vi "Main Loop.vi"(8 "error in (no error)":errorcluster, 10 "Chart Notifier":refnum<notifier>, 11 "Message Queues":T1) -> (0 "error out":errorcluster)   [LabVIEW 2018, in "OPC UA.lvlib" / "OPC UA Module Engine.lvlib"]
uses:
  OPC UA Module Engine.lvlib
  Message Queues.ctl
  support/Message Queue/Message Cluster.ctl
  OPC Display Cluster.ctl
  OPC Module Config.ctl
  Scale Module Folder/Measure Instrument/State Enum.ctl
  <vilib>/Utility/miscctls.llb/LVPoint32TypeDef.ctl
  OPC Settings.ctl
  Variable Data Cluster.ctl
  <vilib>/OPCUA/controls/NodeId.ctl
  <vilib>/OPCUA/controls/OPC UA StatusCode.ctl
  <vilib>/OPCUA/controls/Subscription ID.ctl
  <vilib>/OPCUA/controls/OPC UA Client Refnum.ctl
  <vilib>/OPCUA/controls/Subscription Data Change.ctl
  <vilib>/OPCUA/controls/Data Type.ctl
  <vilib>/Platform/TimedLoop/XDataNode/timing_clust.ctl
  <vilib>/Platform/TimedLoop/XDataNode/nitl_modes.ctl
  <vilib>/Platform/TimedLoop/XDataNode/wakeup.ctl
  Tag VIs/Tag FGV Operation Enum.ctl
  support/Message Queue/Enqueue Message (Single).vi
  <vilib>/Platform/TimedLoop/XDataNode/XDataNode.xnode
  Scale Module Folder/Measure Instrument/Scale Module Engine.lvlib
  OPC UA.lvlib
  <vilib>/Platform/TimedLoop/XDataNode/XDNodeRunTimeDep.lvlib
  support/Support Library.lvlib
  Shared Variables/Dynamic Shared Variables.lvlib
  support/Message Queue/Message Queue.lvlib
panel:
  out "Period (s)":dbl format="%_4g"
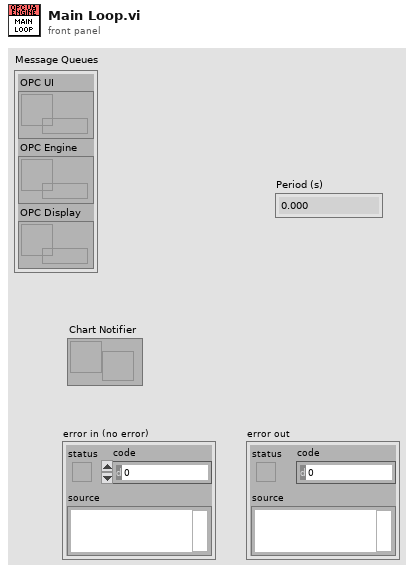
[diagram p1: front panel]
types:
  T1 = typedef "OPC UA.lvlib/Message Queues.ctl" = cluster{"OPC UI":refnum<queue>, "OPC Engine":refnum<queue>, "OPC Display":refnum<queue>}
  T2 = typedef "OPC UA.lvlib/OPC Display Cluster.ctl" = cluster{"URL":string, "Cycle":i32, "Updating":bool}
  T3 = typedef "XDNodeRunTimeDep.lvlib/timing_clust.ctl" = cluster{"Expected End [f-1]":u64, "Actual End [f-1]":u64, "Finished Late? [f-1]":bool, "Expected End [i-1]":u64, "Actual End [i-1]":u64, "Finished Late? [i-1]":bool, "Expected Start [i]":u64, "Actual Start [i]":u64, "Expected Start [f]":u64, "Actual Start [f]":u64, "Source Name":string, "Structure Name":string, "Period":i64, "Deadline":i64, "Offset":i64, "Start":i64, "Priority":i32, "Timeout":i32, "Mode":T4, "Wakeup Reason":T5, "Error":errorcluster, "Source Type":string, "Secondary Source Type":string, "Global End Time":u64, "Global Start Time":u64, "Frame Duration":u64, "Iteration Duration":u64, "Assigned CPU":i32, "I/O Scan Engine Mode":u32}
  T4 = typedef "XDNodeRunTimeDep.lvlib/nitl_modes.ctl" = enum32{"No Change", "Process missed periods, maintain original phase", "Discard missed periods, maintain original phase", "Process missed periods, ignore original phase", "Discard missed periods, ignore original phase"}
  T5 = typedef "XDNodeRunTimeDep.lvlib/wakeup.ctl" = enum32{"Normal", "Aborted", "Asynchronous wakeup", "Timing source error", "Timed loop error", "Timeout"}
  T6 = cluster{"enable? (F)":bool, "name":string, "alarm on":bool, "priority":u32, "ack type":enum16{"Auto", "User", "None", "Each Occurrence"}, "area":string, "description":string, "log? (T)":bool}
  T7 = typedef "Tag FGV Operation Enum.ctl" = enum16{"Init", "Set Notification Queue", "Create Tag", "Commit", "Write Tag (Numeric)", "Write Tag (Boolean)", "Read All Tags", "Read One Tag", "Delete Tag Category", "Set Alarm Parameters (Numeric)", "Set Alarm Parameters (Boolean)", "Enable All Alarms", "Disable All Alarms", "Delete All Tags", "Read Alarms", "Ack Alarm", "Read Alarm Parameters (Numeric)", "Read Alarm Parameters (Boolean)"}
  T8 = enum32{"u32BitField", "bool", "double", "string", "int8", "uint8", "int16", "uint16", "int32", "uint32", "int64", "uint64", "single", "double waveform", "int16 waveform", "array of boolean", "array of int8", "array of uint8", "array of int16", "array of uint16", "array of int32", "array of uint32", "array of int64", "array of uint64", "array of single", "array of double", "array of double waveform", "array of int16 waveform", "array of string", "variant", "timestamp", "fixed point", "custom"}
  T9 = typedef "Scale Module.lvlib/Scale Module Engine.lvlib/State Enum.ctl" = enum16{"Measuring", "Idle"}
  T10 = typedef "OPC UA.lvlib/OPC Settings.ctl" = cluster{"Cycle Period":dbl, "server endpoint URL":string, "security policy":cluster{"message mode":enum16{"None", "Sign", "Sign and Encrypt"}, "security":enum16{"Basic256", "Basic128Rsa15"}}, "Trust Any Server":bool}
  T11 = typedef "OPC UA.lvlib/OPC Module Config.ctl" = cluster{"State":T9, "GUID":string, "Drop Coords":T12, "Configuration":T10, "First Iteration":bool, "Data":cluster{"Object Name":string, "Variable Array":T13[]}[], "Process Name":string, "Load Count":i32, "Log Started":bool, "subscription ID out":T16, "OPC UA client refnum out":T17, "Event Registration Refnum":refnum<event-registration>, "Start Time":timestamp, "Current Time":timestamp}
  T12 = typedef "LVPoint32TypeDef.ctl" = cluster{"Horizontal":i32, "Vertical":i32}
  T13 = typedef "OPC UA.lvlib/Variable Data Cluster.ctl" = cluster{"node ID":T14, "browse name":string, "status":T15, "timestamp":timestamp, "value ":variant}
  T14 = typedef "NodeId.ctl" = string
  T15 = typedef "OPC UA StatusCode.ctl" = u32
  T16 = typedef "Subscription ID.ctl" = u32
  T17 = typedef "OPC UA Client Refnum.ctl" = refnum<k21>
  T18 = cluster{"Object Name":string, "Variable Array":T13[]}[]
  T19 = cluster{"Object Name":string, "Variable Array":T13[]}
  T20 = typedef "Support Library.lvlib/Message Queue.lvlib/Message Cluster.ctl" = cluster{"Message":string, "Message Data":variant}
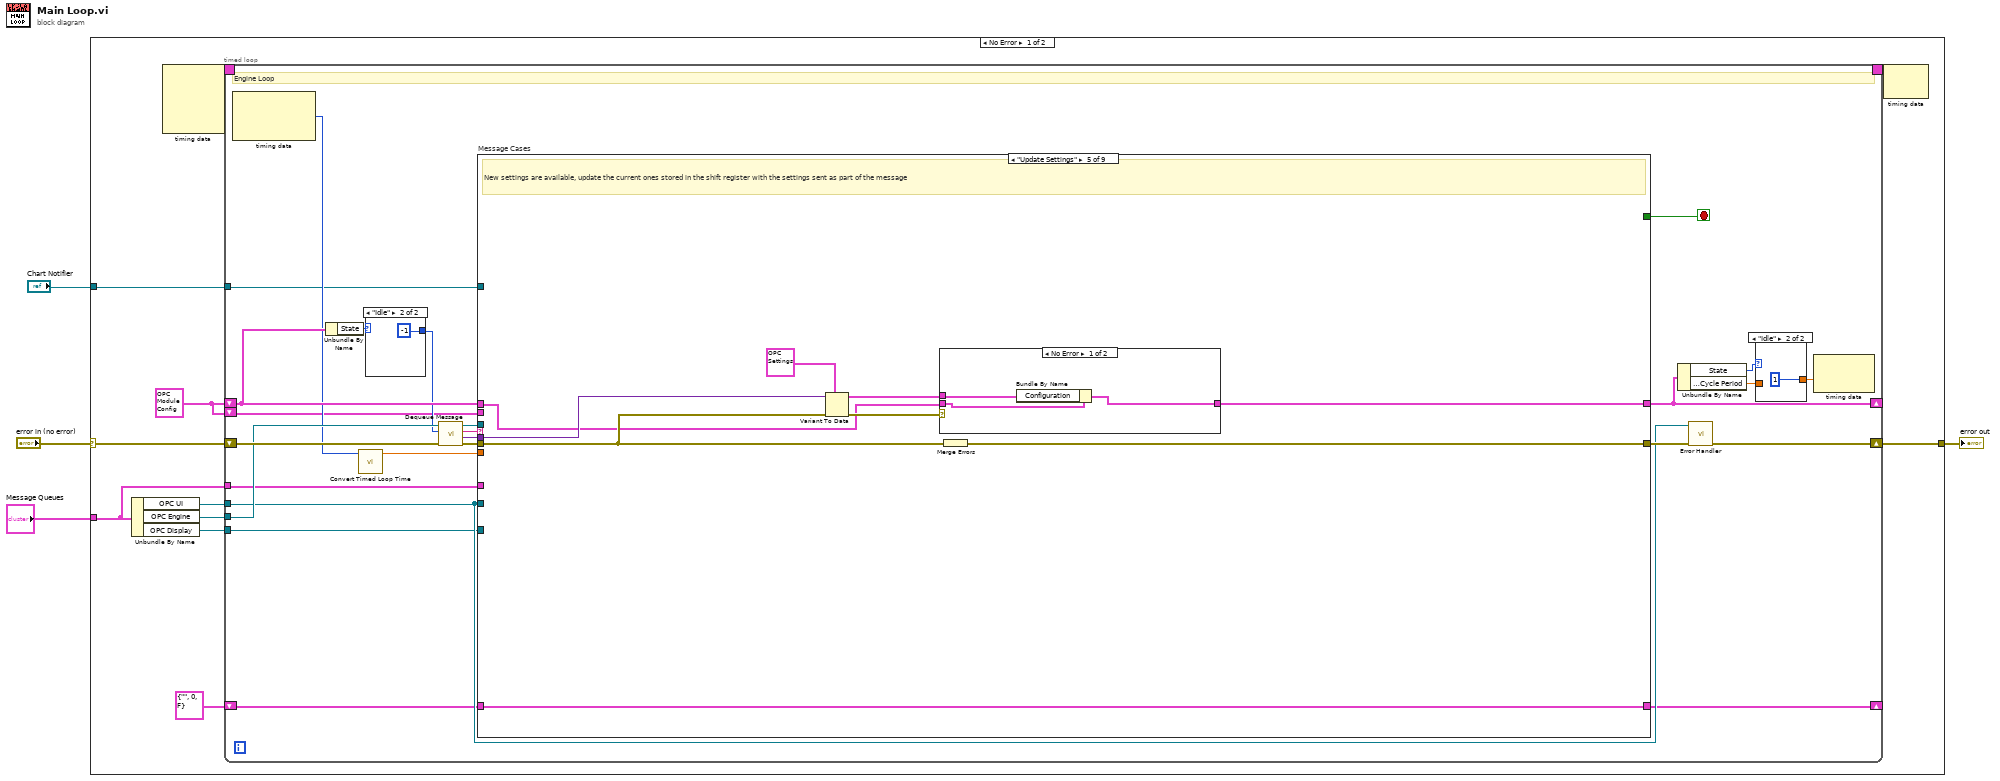
[diagram p0: block diagram]
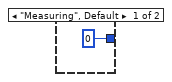
[diagram p3: hidden frame]
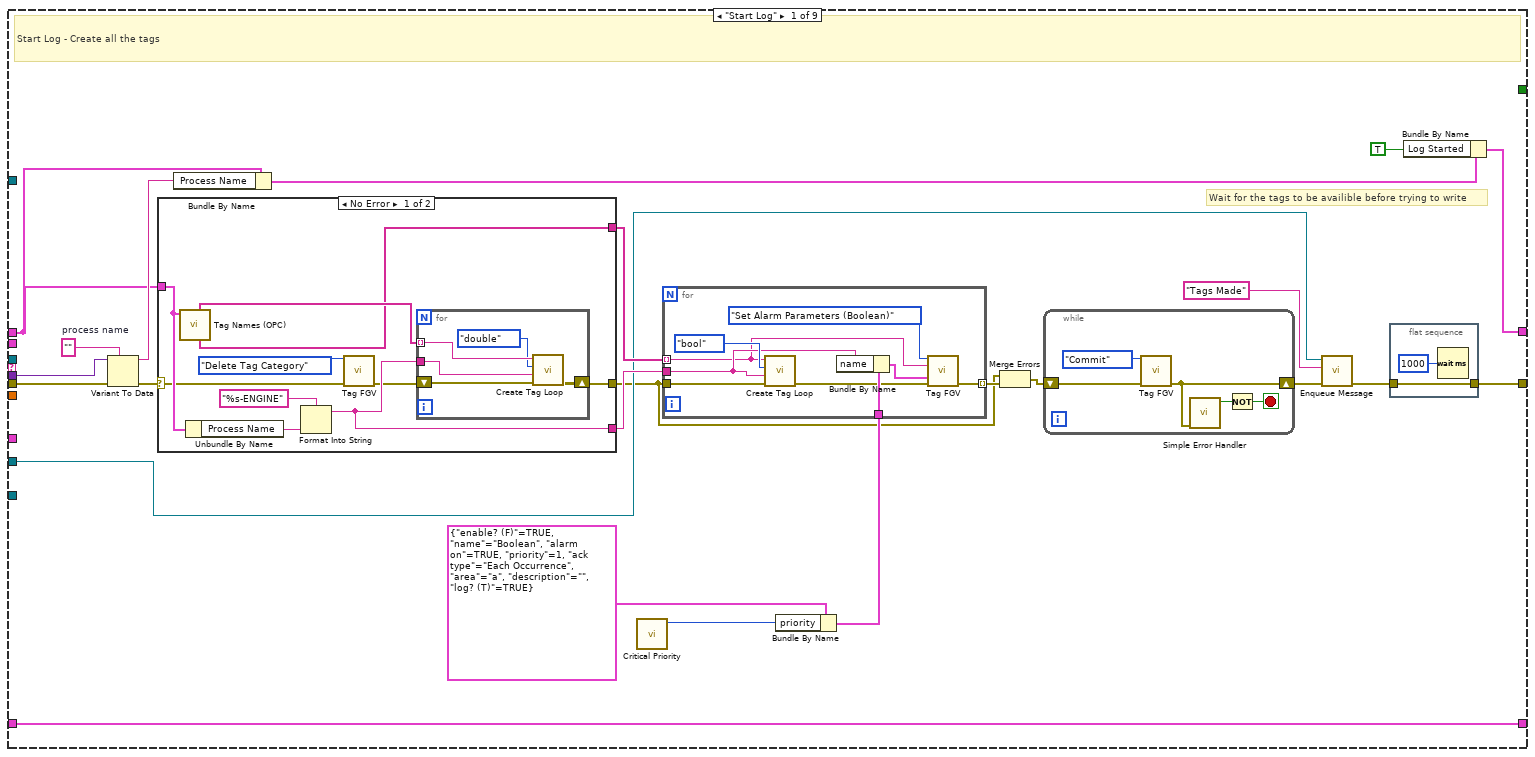
[diagram p4: hidden frame]
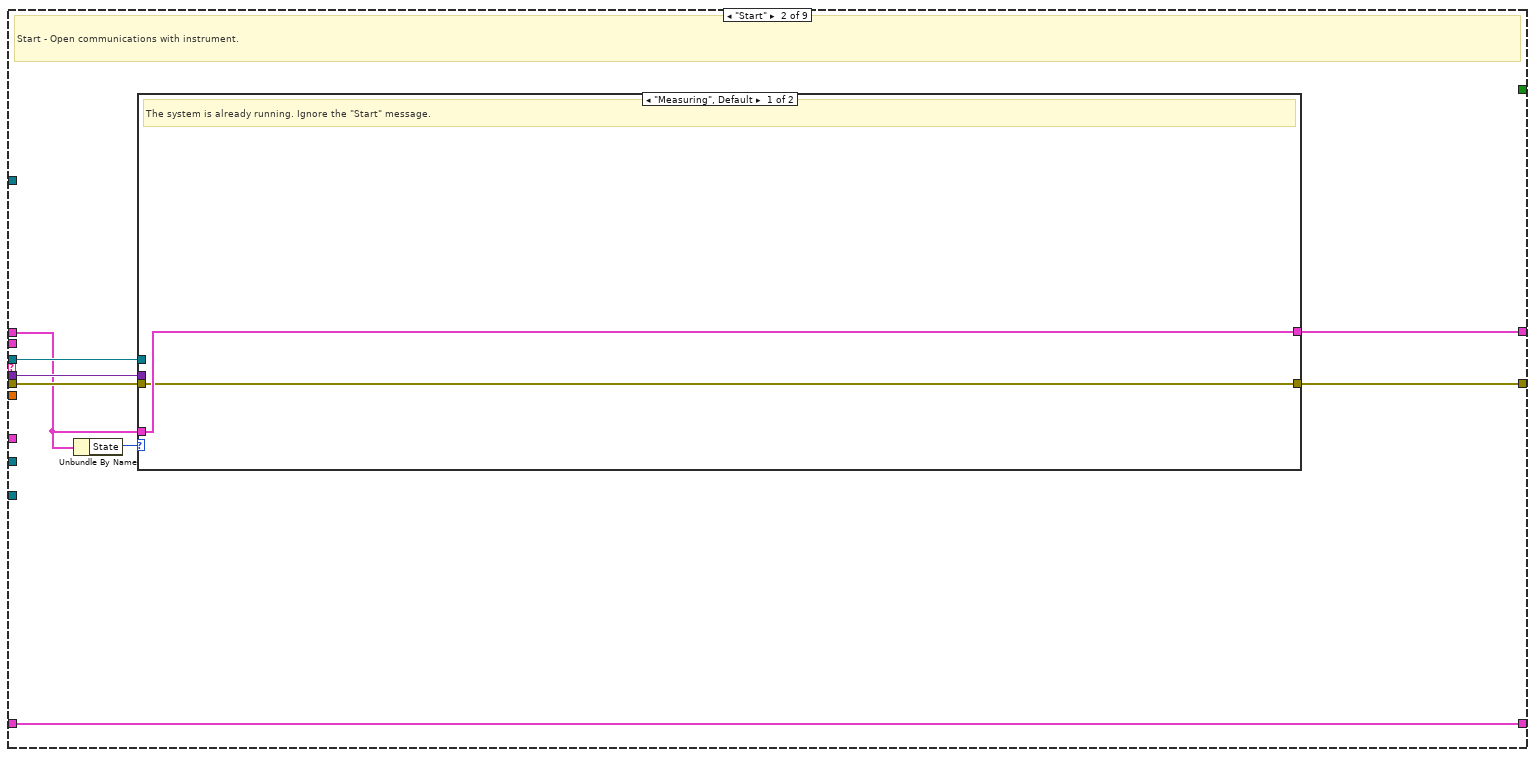
[diagram p6: hidden frame]
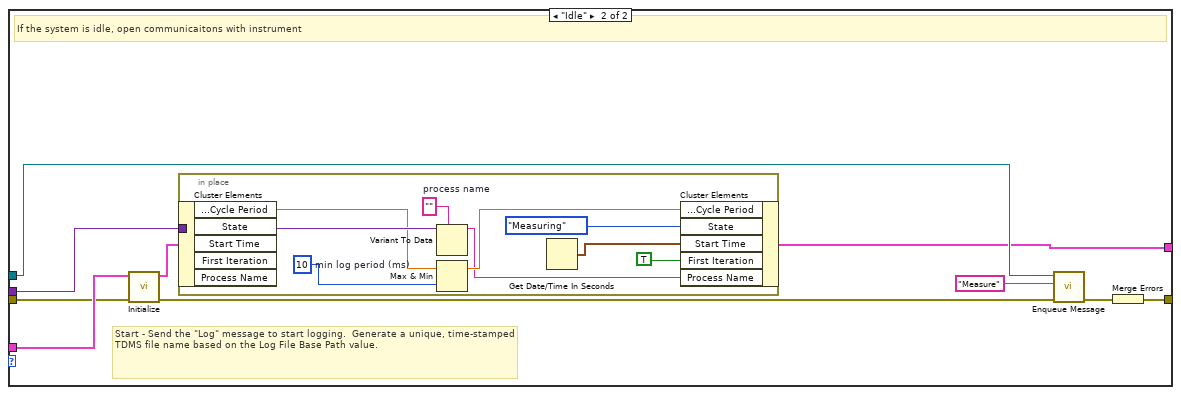
[diagram p7: hidden frame]
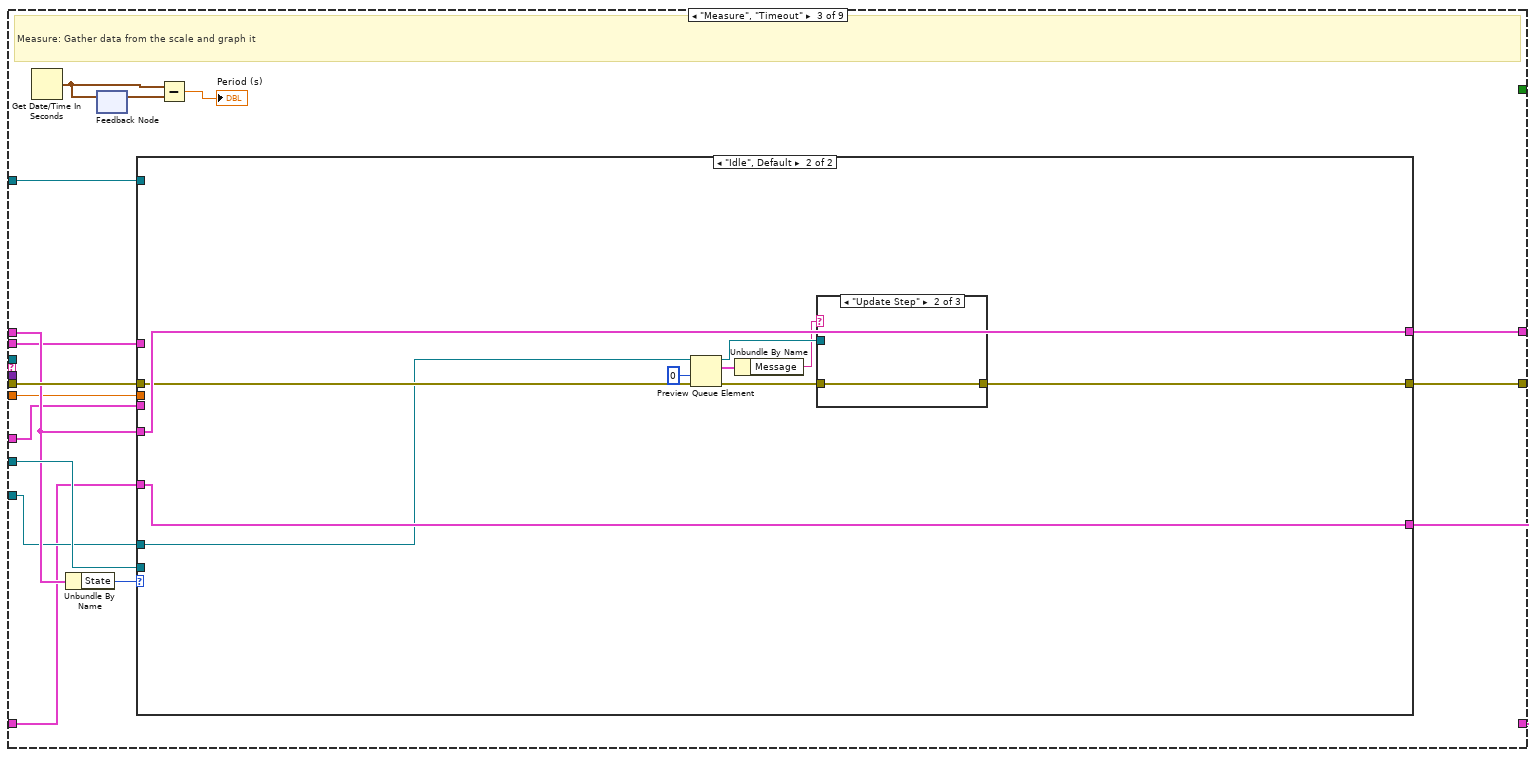
[diagram p8: hidden frame]
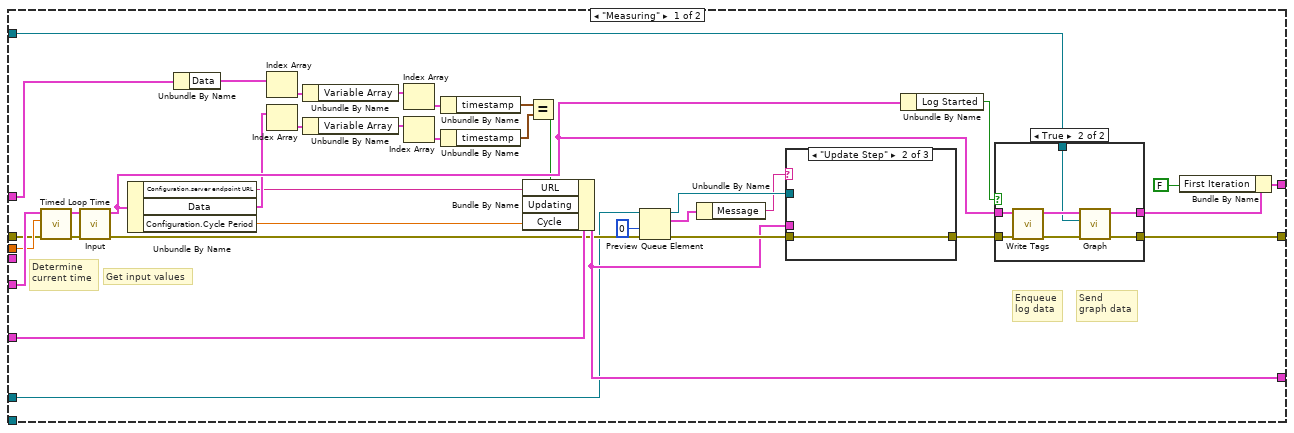
[diagram p9: hidden frame]
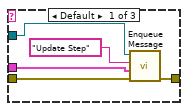
[diagram p10: hidden frame]
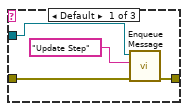
[diagram p13: hidden frame]
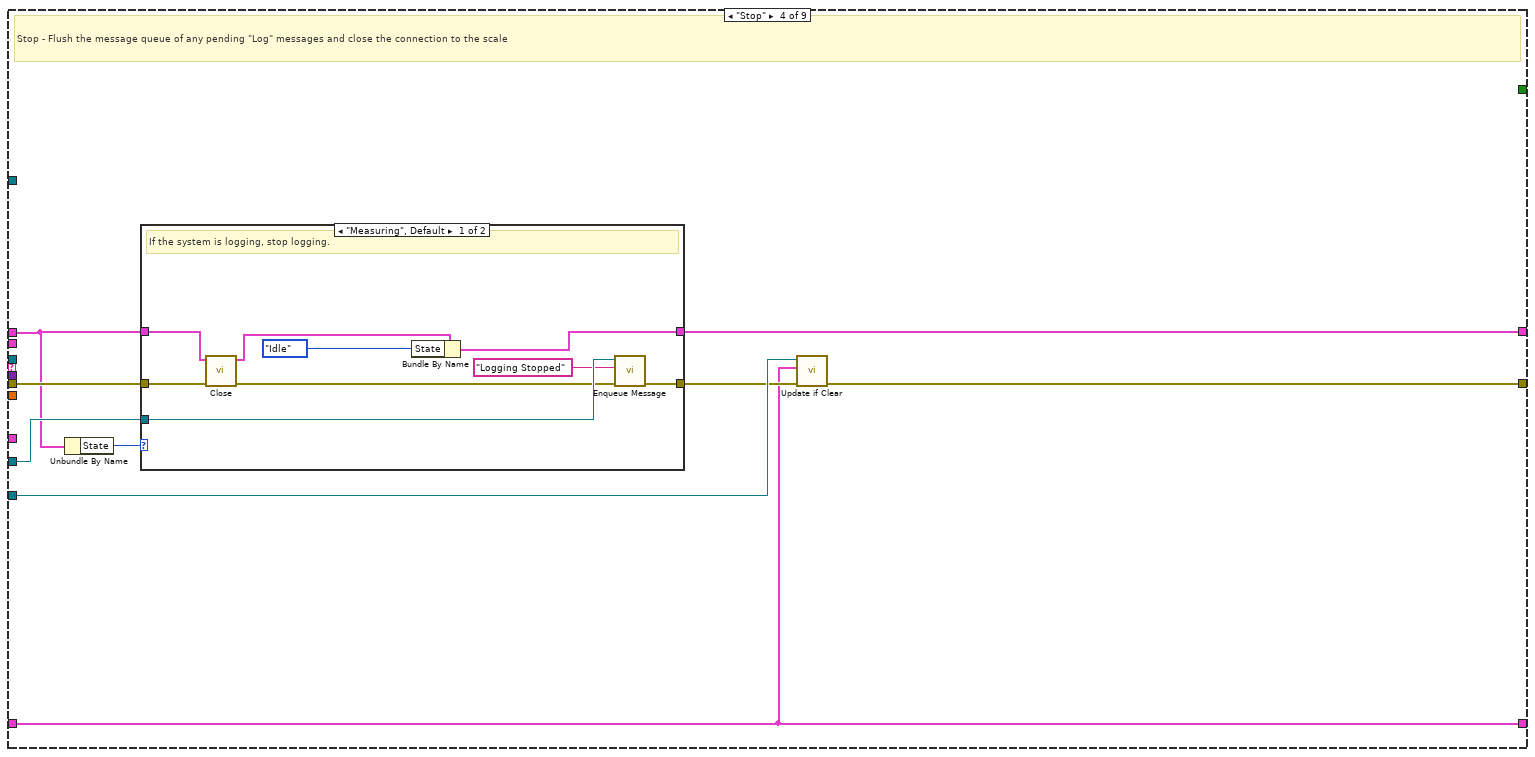
[diagram p15: hidden frame]
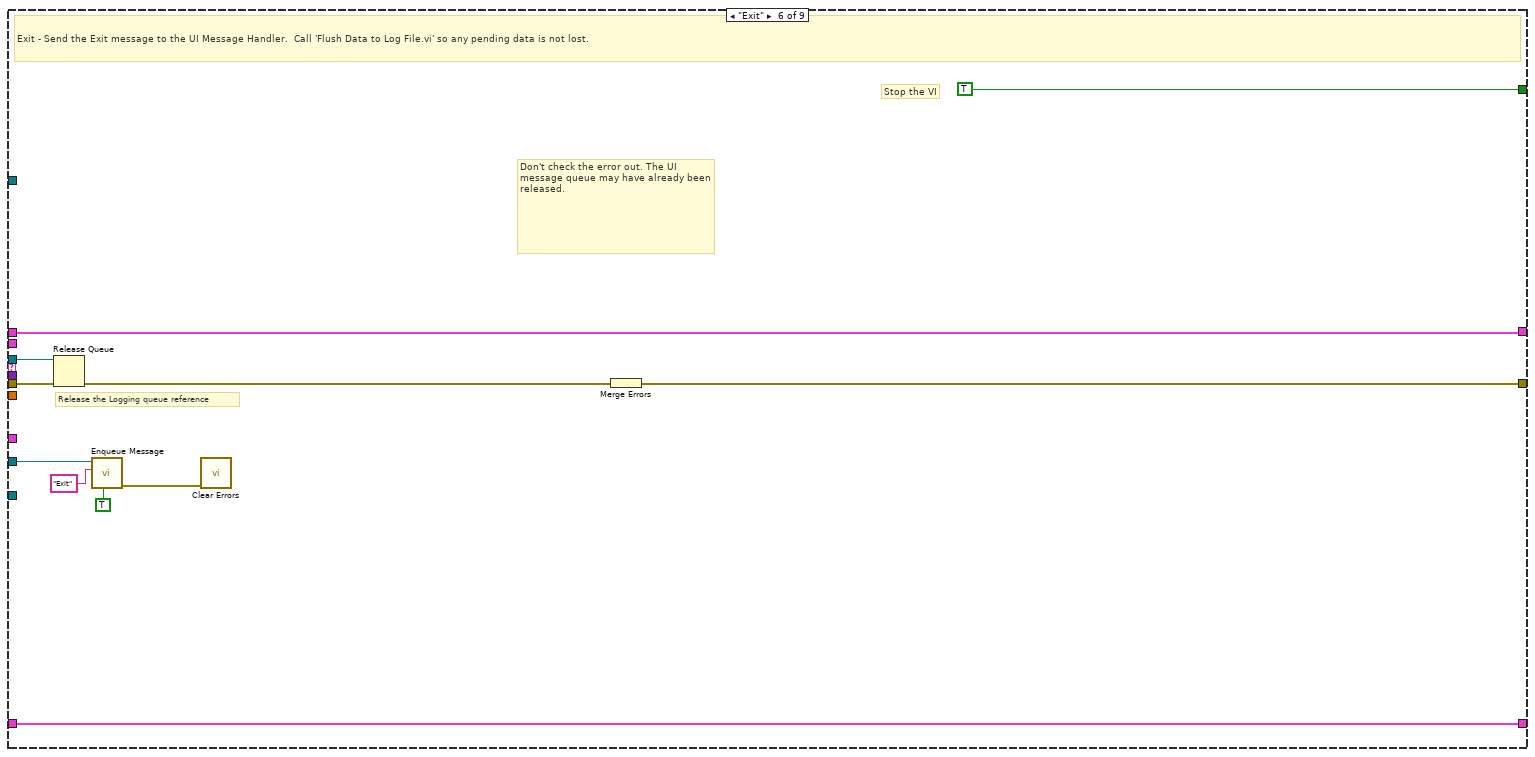
[diagram p18: hidden frame]
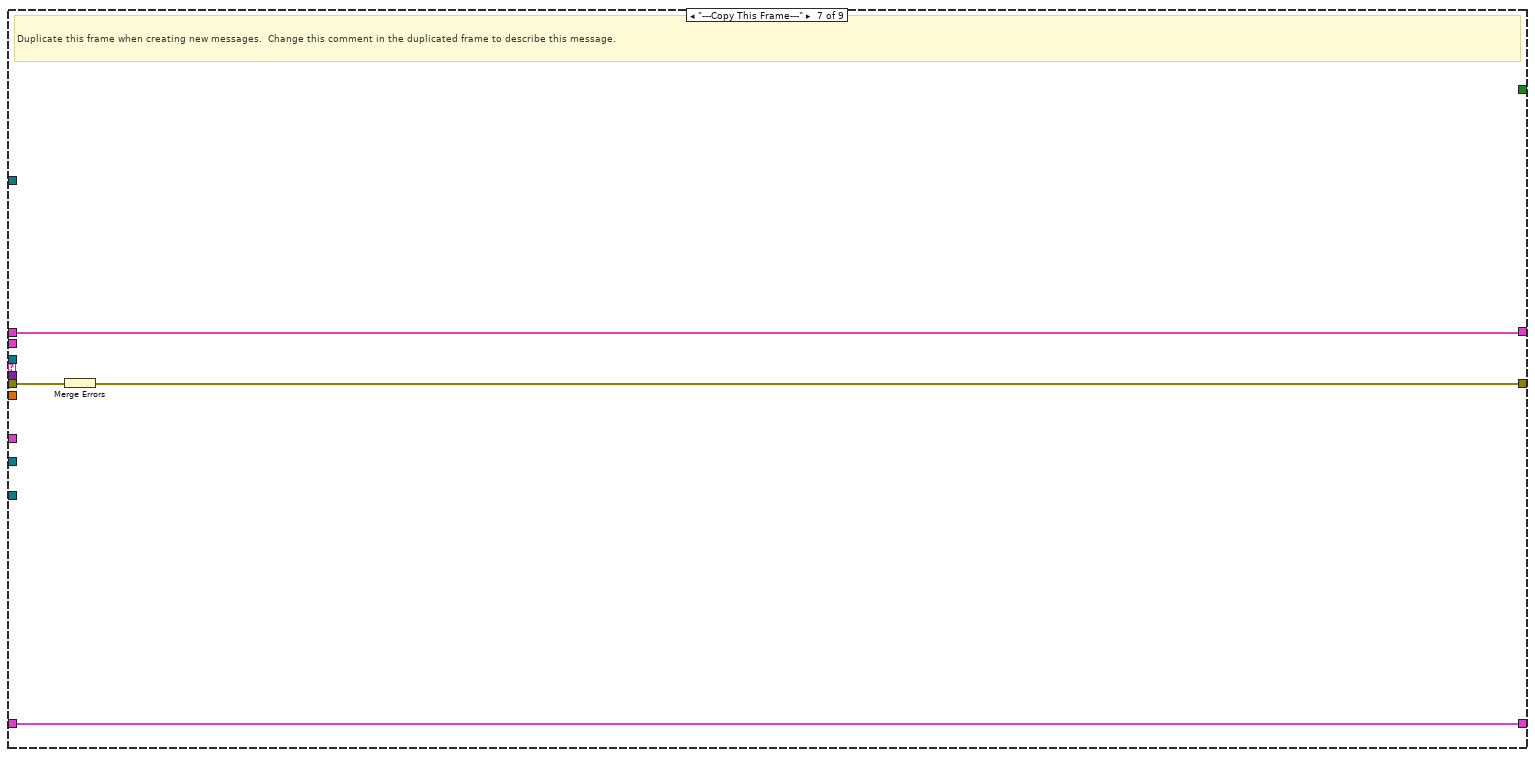
[diagram p19: hidden frame]
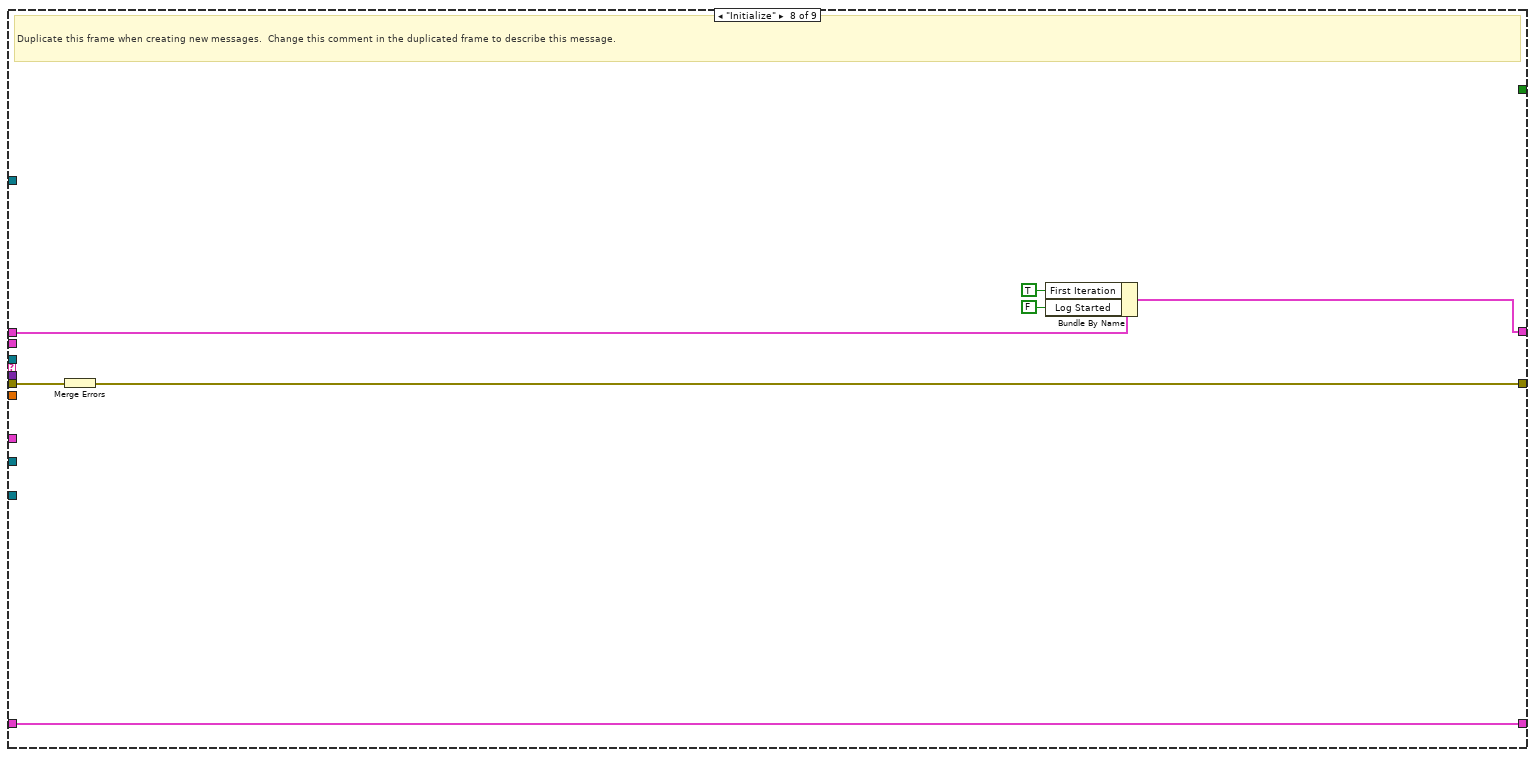
[diagram p20: hidden frame]
diagram:
  n1 = case shown="No Error" "error in (no error)" {
    selector: "error in (no error)" -> [w14 w283]
    tunnel: "Message Queues" -> [w10 _]
    tunnel: [w15 w283] -> w4
    tunnel: "Chart Notifier" -> [w8 _]
    frame No Error {
      w5 = T11 {"State"=enum."Idle", "GUID"="", "Drop Coords"={"Horizontal"=0, "Vertical"=0}, "Configuration"={"Cycle Period"=500.0, "server endpoint URL"="opc.tcp://10.131.1.22:4840", "security policy"={"message mode"=enum."None", "security"=enum."Basic256"}, "Trust Any Server"=FALSE}, "First Iteration"=FALSE, "Data"=[], "Process Name"="", "Load Count"=0, "Log Started"=FALSE, "subscription ID out"=0, "OPC UA client refnum out"="", "Event Registration Refnum"=refnum, "Start Time"=timestamp(0 s since 1904-01-01), "Current Time"=timestamp(0 s since 1904-01-01)} ("OPC Module Config")
      n2 = Unbundle By Name(w10) -> ("OPC UI"=w13:refnum<queue>, "OPC Engine"=w9:refnum<queue>, "OPC Display"=w7:refnum<queue>)
      n3 = node-c288() -> (w12:T3)  [unwired: 4 in]
      n4 = timed-loop {
        tunnel: w9 -> [w34]
        shift-right: [w18] -> _
        shift-left: w5 -> [w30]
        shift-right: [w32] -> w15
        shift-left: w14 -> [w39]
        tunnel: w13 -> [w31]
        timing: w12 -> [_]
        timing-out: [_] -> w11
        tunnel: w10 -> [w22]
        tunnel: w8 -> [w21]
        tunnel: w7 -> [w20]
        shift-right: [w19] -> _
        shift-left: T2 {"URL"="", "Cycle"=0, "Updating"=FALSE} ("OPC Display Cluster") -> [w17]
        shift-left: w5 -> [w16]
        stop <- w40 stop-if-true
        # "Engine Loop"
        n5 = node-c288() -> (w24:i64)  [unwired: 1 in, 2 out]
        n6 = Unbundle By Name(w30) -> ("State"=w29:T9)
        n7 = call "Convert Timed Loop Time.vi"("Actual Start [i]"=w24) -> ("ET since start (s)"=w23:dbl)  [unwired: 10 in]
        n8 = case shown="\"Idle\"" w29 {
          tunnel: [0 ("timeout in ms (-1)") -1 ("timeout in ms (-1)")] -> w28
          frame "Measuring", Default {
          }
          frame "Idle" {
          }
        }
        n9 = call "Dequeue Message.vi"("error in (no error)"=w39, "timeout in ms (-1)"=w28, "Message Queue"=w34) -> ("error out"=w38:errorcluster, "Message Data"=w36:variant, "Message"=w37:string, "dup Message Queue"=w35:refnum<queue>)  [unwired: 5 in]
        n10 = case "Message Cases" shown="\"Update Settings\"" w37 {
          selector: w37 -> [_ _ _ _ _ _ _ _ w274]
          tunnel: w35 -> [_ w111 _ _ _ w255 _ _ _]
          tunnel: w38 -> [w67 w110 w146 w226 w244 w258 w265 w272 _]
          tunnel: [w51 w112 w147 w218 w246 w260 w264 w271 w273] -> w33
          tunnel: w30 -> [w53 w107 w145 w223 w242 w251 w262 w269 w279]
          tunnel: [_ _ _ _ _ TRUE _ _ _] -> w40
          tunnel: w36 -> [w68 w108 _ _ w245 _ _ _ _]
          tunnel: w31 -> [w56 _ w148 w225 _ w259 _ _ _]
          tunnel: w23 -> [_ _ w144 _ _ _ _ _ _]
          tunnel: w22 -> [_ _ w143 _ _ _ _ _ _]
          tunnel: w21 -> [_ _ w139 _ _ _ _ _ _]
          tunnel: w20 -> [_ _ w138 w221 _ _ _ _ _]
          tunnel: w17 -> [w72 w106 w137 w219 w240 w252 w263 w270 w280]
          tunnel: [w72 w106 w136 w219 w240 w252 w263 w270 w280] -> w19
          tunnel: [w59 w105 w135 w222 w239 w251 w262 w266 w279] -> w18
          tunnel: w16 -> [_ _ w134 _ _ _ _ _ _]
          frame "Start Log" {
            w71 = ""  # process name
            # "Wait for the tags to be availible before trying to write"
            # "Start Log - Create all the tags"
            n11 = Variant To Data(error in=w67, type=w71, Variant=w68) -> (data=w69:string, error out=w70:errorcluster)
            n12 = case shown="No Error" w70 {
              selector: w70 -> [w90 w104]
              tunnel: [w98 w104] -> w50
              tunnel: [w96 _] -> w63
              tunnel: [w94 _] -> w62
              tunnel: w53 -> [w93 _]
              frame No Error {
                n13 = call "Tag Names (OPC).vi"("OPC Module Config"=w93) -> ("All Boolean Tags"=w94:string[], "All  Numeric Tags"=w95:string[])  [unwired: 8 in, 1 out]
                n14 = Unbundle By Name(w93) -> ("Process Name"=w92:string)
                n15 = Format Into String(format string="%s-ENGINE", w92) -> (resulting string=w96:string)  [unwired: 2 in, 1 out]
                n16 = call "Tag FGV.vi"("Operation"=Tag_FGV_Operation_Enum."Delete Tag Category", "error in (no error)"=w90) -> ("error out"=w89:errorcluster)  [unwired: 6 in, 7 out]
                n17 = for {
                  shift-right: [w103] -> w98
                  shift-left: w89 -> [w102]
                  tunnel: w96 -> [w99]
                  tunnel: w95 -> [w101] mode=indexing
                  n18 = call "Create Tag Loop.vi"("error in (no error)"=w102, "Tag Category"=w99, "data type"=T8."double", "Tag Name"=w101) -> ("error out"=w103:errorcluster)  [unwired: 7 in]
                }
              }
              frame Error {
              }
            }
            n19 = Bundle By Name(cluster=w53, "Process Name"=w69) -> (w60:T11)
            n20 = call "Critical Priority.vi"() -> ("critical priority"=w65:i32)  [unwired: 11 in]
            n21 = Bundle By Name(cluster=T6 {"enable? (F)"=TRUE, "name"="Boolean", "alarm on"=TRUE, "priority"=1, "ack type"=enum."Each Occurrence", "area"="a", "description"="", "log? (T)"=TRUE} ("Boolean alarm settings"), "priority"=w65) -> (w64:T6)
            n22 = for {
              tunnel: w64 -> [w88]
              tunnel: [w80] -> w61 mode=indexing
              tunnel: w62 -> [w83] mode=indexing
              tunnel: w63 -> [w85]
              tunnel: w50 -> [w87]
              n23 = call "Create Tag Loop.vi"("error in (no error)"=w87, "Tag Category"=w85, "data type"=T8."bool", "Tag Name"=w83) -> ("error out"=w81:errorcluster)  [unwired: 7 in]
              n24 = Bundle By Name(cluster=w88, "name"=w85) -> (w82:T6)
              n25 = call "Tag FGV.vi"("Operation"=Tag_FGV_Operation_Enum."Set Alarm Parameters (Boolean)", "Tag Name"=w83, "Data"=w82, "error in (no error)"=w81) -> ("error out"=w80:errorcluster)  [unwired: 4 in, 7 out]
            }
            n26 = Merge Errors(w50, w61) -> (w54:errorcluster)
            n27 = while {
              shift-right: [w75] -> w55
              shift-left: w54 -> [w76]
              stop <- w78 stop-if-true
              n28 = call "Tag FGV.vi"("Operation"=Tag_FGV_Operation_Enum."Commit", "error in (no error)"=w76) -> ("error out"=w75:errorcluster)  [unwired: 6 in, 7 out]
              n29 = call <vilib>:"Simple Error Handler.vi"("error in (no error)"=w75) -> ("error?"=w79:bool)  [unwired: 4 in, 4 out]
              n30 = Not(x=w79) -> (.not. x?=w78:bool)
            }
            n31 = call-poly "Enqueue Message.vi"("error in (no error)"=w55, "Message"="Tags Made", "Message Queue"=w56) -> ("error out"=w52:errorcluster)  [unwired: 7 in, 1 out]
            n32 = flat-sequence {
              tunnel: [w73] -> w51
              tunnel: w52 -> [w73]
              frame #0 {
                n33 = Wait (ms)(milliseconds to wait=u32 1000) -> ()  [unwired: 1 out]
              }
            }
            n34 = Bundle By Name(cluster=w60, "Log Started"=TRUE) -> (w59:T11)
          }
          frame "Start" {
            # "Start - Open communications with instrument."
            n35 = Unbundle By Name(w107) -> ("State"=w109:T9)
            n36 = case shown="\"Measuring\", Default" w109 {
              tunnel: [w113 w124] -> w112
              tunnel: w111 -> [_ w121]
              tunnel: w110 -> [w113 w118]
              tunnel: w107 -> [w114 w119]
              tunnel: [w114 w115] -> w105
              tunnel: w108 -> [_ w120]
              frame "Measuring", Default {
                # "The system is already running. Ignore the \"Start\" message."
              }
              frame "Idle" {
                # "Start - Send the \"Log\" message to start logging.  Generate a unique, time-stamped TDMS file name based on the Log File Base Path value."
                # "If the system is idle, open communicaitons with instrument"
                n37 = call "Initialize.vi"("error in"=w118, "OPC Module Config In"=w119) -> ("error out"=w117:errorcluster, "OPC Module Config Out"=w116:T11)  [unwired: 8 in]
                n38 = in-place {
                  in-place-border: w120 -> [w131]
                  w132 = ""  # process name
                  w133 = 10  # min log period (ms)
                  n39 = in-place-cluster #1(w116) -> ("Configuration.Cycle Period"=w130:dbl)  [unwired: 4 out]
                  n40 = Variant To Data(type=w132, Variant=w131) -> (data=w125:string)  [unwired: 1 in, 1 out]
                  n41 = Max & Min(x=w130, y=w133) -> (max(x,y)=w129:dbl)  [unwired: 1 out]
                  n42 = Get Date/Time In Seconds() -> (seconds since 1Jan1904=w127:timestamp)
                  n43 = in-place-cluster #1("Configuration.Cycle Period"=w129, "State"=State_Enum."Measuring", "Start Time"=w127, "First Iteration"=TRUE, "Process Name"=w125) -> (w115:T11)
                }
                n44 = call-poly "Enqueue Message.vi"("error in (no error)"=w117, "Message"="Measure", "Message Queue"=w121) -> ("error out"=w122:errorcluster)  [unwired: 7 in, 1 out]
                n45 = Merge Errors(w122) -> (w124:errorcluster)
              }
            }
          }
          frame "Measure", "Timeout" {
            # "Measure: Gather data from the scale and graph it"
            n46 = Get Date/Time In Seconds() -> (seconds since 1Jan1904=w141:timestamp)
            n47 = Unbundle By Name(w145) -> ("State"=w149:T9)
            n48 = feedback-in #2(w141) -> ()
            n49 = feedback #2() -> (w142:timestamp)  [unwired: 1 in]
            n50 = case shown="\"Idle\", Default" w149 {
              tunnel: w146 -> [w175 w204]
              tunnel: w145 -> [w177 w210]
              tunnel: w148 -> [_ _]
              tunnel: [w185 w202] -> w147
              tunnel: [w183 w210] -> w135
              tunnel: w144 -> [w176 _]
              tunnel: w143 -> [_ _]
              tunnel: w139 -> [w181 _]
              tunnel: w138 -> [w151 w203]
              tunnel: w137 -> [w180 w211]
              tunnel: [w153 w211] -> w136
              tunnel: w134 -> [w171 _]
              frame "Measuring" {
                # "Determine\ncurrent time"
                # "Send\ngraph data"
                # "Enqueue\nlog data"
                # "Get input values"
                n51 = call "Timed Loop Time.vi"("error in (no error)"=w175, "ET since start (s)"=w176, "OPC Module Config In"=w177) -> ("error out"=w173:errorcluster, "OPC Module Config Out"=w174:T11)  [unwired: 7 in]
                n52 = call "Input.vi"("error in"=w173, "OPC Module Config In"=w174) -> ("error out"=w152:errorcluster, "OPC Module Config Out"=w172:T11)  [unwired: 8 in]
                n53 = Unbundle By Name(w172) -> ("Configuration.server endpoint URL"=w159:string, "Data"=w163:T18, "Configuration.Cycle Period"=w179:dbl)
                n54 = Unbundle By Name(w171) -> ("Data"=w170:T18)
                n55 = Index Array(array=w170) -> (element=w169:T19)  [unwired: 1 in]
                n56 = Index Array(array=w163) -> (element=w164:T19)  [unwired: 1 in]
                n57 = Unbundle By Name(w169) -> ("Variable Array"=w168:T13[])
                n58 = Unbundle By Name(w164) -> ("Variable Array"=w165:T13[])
                n59 = Index Array(array=w168) -> (element=w167:T13)  [unwired: 1 in]
                n60 = Index Array(array=w165) -> (element=w166:T13)  [unwired: 1 in]
                n61 = Unbundle By Name(w167) -> ("timestamp"=w162:timestamp)
                n62 = Unbundle By Name(w166) -> ("timestamp"=w161:timestamp)
                n63 = Equal?(x=w162, y=w161) -> (x = y?=w160:bool)
                n64 = Bundle By Name(cluster=w180, "URL"=w159, "Updating"=w160, "Cycle"=w179) -> (w153:T2)
                n65 = Preview Queue Element(queue=w151, timeout in ms (-1)=0, error in (no error)=w152) -> (queue out=w157:refnum<queue>, element=w156:T20, error out=w154:errorcluster)  [unwired: 1 out]
                n66 = Unbundle By Name(w156) -> ("Message"=w155:string)
                n67 = case shown="\"Update Step\"" w155 {
                  tunnel: w153 -> [w186 _ _]
                  tunnel: w157 -> [w187 _ _]
                  tunnel: [w188 w191 w192] -> w150
                  tunnel: w154 -> [w189 w191 w192]
                  frame Default {
                    n68 = call-poly "Enqueue Message.vi"("error in (no error)"=w189, "Message Data"=w186, "Message"="Update Step", "Message Queue"=w187) -> ("error out"=w188:errorcluster)  [unwired: 6 in, 1 out]
                  }
                  frame "Update Step" {
                  }
                  frame "Exit" {
                  }
                }
                n69 = Unbundle By Name(w172) -> ("Log Started"=w178:bool)
                n70 = case shown="True" w178 {
                  tunnel: [w193 w195] -> w185
                  tunnel: [w194 w196] -> w184
                  tunnel: w181 -> [_ w198]
                  tunnel: w172 -> [w194 w201]
                  tunnel: w150 -> [w193 w200]
                  frame False {
                  }
                  frame True {
                    n71 = call "Write Tags.vi"("error in (no error)"=w200, "OPC Module Config In"=w201) -> ("error out"=w197:errorcluster, "OPC Module Config Out"=w199:T11)  [unwired: 8 in]
                    n72 = call "Graph.vi"("error in (no error)"=w197, "notifier out"=w198, "OPC Module Config In"=w199) -> ("error out"=w195:errorcluster, "OPC Module Config Out"=w196:T11)  [unwired: 7 in]
                  }
                }
                n73 = Bundle By Name(cluster=w184, "First Iteration"=FALSE) -> (w183:T11)
              }
              frame "Idle", Default {
                n74 = Preview Queue Element(queue=w203, timeout in ms (-1)=0, error in (no error)=w204) -> (queue out=w208:refnum<queue>, element=w207:T20, error out=w205:errorcluster)  [unwired: 1 out]
                n75 = Unbundle By Name(w207) -> ("Message"=w206:string)
                n76 = case shown="\"Update Step\"" w206 {
                  tunnel: w208 -> [w212 _ _]
                  tunnel: [w213 w216 w217] -> w202
                  tunnel: w205 -> [w214 w216 w217]
                  frame Default {
                    n77 = call-poly "Enqueue Message.vi"("error in (no error)"=w214, "Message"="Update Step", "Message Queue"=w212) -> ("error out"=w213:errorcluster)  [unwired: 7 in, 1 out]
                  }
                  frame "Update Step" {
                  }
                  frame "Exit" {
                  }
                }
              }
            }
            n78 = Subtract(x=w141, y=w142) -> (x-y=→"Period (s)":dbl)
          }
          frame "Stop" {
            # "Stop - Flush the message queue of any pending \"Log\" messages and close the connection to the scale"
            n79 = Unbundle By Name(w223) -> ("State"=w224:T9)
            n80 = case shown="\"Measuring\", Default" w224 {
              tunnel: [w231 w237] -> w220
              tunnel: w226 -> [w229 w237]
              tunnel: w225 -> [w235 _]
              tunnel: w223 -> [w230 w236]
              tunnel: [w233 w236] -> w222
              frame "Measuring", Default {
                # "If the system is logging, stop logging."
                n81 = call "Close.vi"("error in"=w229, "OPC Module Config In"=w230) -> ("error out"=w227:errorcluster, "OPC Module Config Out"=w228:T11)  [unwired: 8 in]
                n82 = Bundle By Name(cluster=w228, "State"=State_Enum."Idle") -> (w233:T11)
                n83 = call-poly "Enqueue Message.vi"("error in (no error)"=w227, "Message"="Logging Stopped", "Message Queue"=w235) -> ("error out"=w231:errorcluster)  [unwired: 7 in, 1 out]
              }
              frame "Idle" {
                # "The system is already idle. Ignore the \"Stop\" message."
              }
            }
            n84 = call "Update if Clear.vi"("error in (no error)"=w220, "Message Data"=w219, "Queue in"=w221) -> ("error out"=w218:errorcluster)  [unwired: 8 in]
          }
          frame "Update Settings" {
            # "New settings are available, update the current ones stored in the shift register with the settings sent as part of the message"
            n85 = Variant To Data(error in=w244, type=T10 {"Cycle Period"=500.0, "server endpoint URL"="opc.tcp://10.131.1.22:4840", "security policy"={"message mode"=enum."Sign", "security"=enum."Basic256"}, "Trust Any Server"=FALSE} ("OPC Settings"), Variant=w245) -> (data=w241:T10, error out=w243:errorcluster)
            n86 = case shown="No Error" w243 {
              tunnel: w242 -> [w249 w250]
              tunnel: w241 -> [w248 _]
              tunnel: [w247 w250] -> w239
              frame No Error {
                n87 = Bundle By Name(cluster=w249, "Configuration"=w248) -> (w247:T11)
              }
              frame Error {
              }
            }
            n88 = Merge Errors(w244) -> (w246:errorcluster)
          }
          frame "Exit" {
            # "Release the Logging queue reference"
            # "Don't check the error out. The UI message queue may have already been released."
            # "Stop the VI"
            # "Exit - Send the Exit message to the UI Message Handler.  Call 'Flush Data to Log File.vi' so any pending data is not lost."
            n89 = Release Queue(queue=w255, error in (no error)=w258) -> (error out=w254:errorcluster)  [unwired: 1 in, 2 out]
            n90 = call-poly "Enqueue Message.vi"("Priority Message? (F)"=TRUE, "Message"="Exit", "Message Queue"=w259) -> ("error out"=w253:errorcluster)  [unwired: 7 in, 1 out]
            n91 = call <vilib>:"Clear Errors.vi"("error in (no error)"=w253) -> ()  [unwired: 5 in, 2 out]
            n92 = Merge Errors(w254) -> (w260:errorcluster)
          }
          frame "---Copy This Frame---" {
            # "Duplicate this frame when creating new messages.  Change this comment in the duplicated frame to describe this message."
            n93 = Merge Errors(w265) -> (w264:errorcluster)
          }
          frame "Initialize" {
            # "Duplicate this frame when creating new messages.  Change this comment in the duplicated frame to describe this message."
            n94 = Merge Errors(w272) -> (w271:errorcluster)
            n95 = Bundle By Name(cluster=w269, "First Iteration"=TRUE, "Log Started"=FALSE) -> (w266:T11)
          }
          frame Default {
            # "'Default' case only runs if there is a message that isn't defined in any of the other cases.  Output a programming error."
            n96 = Concatenate Strings("The invalid message string " ("string"), w274, " was received in the OPC UA Engine." ("string")) -> (w275:string)
            n97 = Bundle By Name(cluster=errorcluster {"status"=TRUE, "code"=1, "source"=""} ("error constant"), "source"=w275) -> (w273:errorcluster)
          }
        }
        n98 = Unbundle By Name(w18) -> ("State"=w27:T9, "Configuration.Cycle Period"=w25:dbl)
        n99 = call "Error Handler.vi"("error in (no error)"=w33, "Message Queue"=w31) -> ("dup error in"=w32:errorcluster)  [unwired: 8 in, 1 out]
        n100 = case shown="\"Idle\"" w27 {
          tunnel: [w41 1] -> w26
          tunnel: w25 -> [w41 _]
          frame "Measuring" {
          }
          frame "Idle" {
          }
        }
        n101 = node-c288(w26) -> ()  [unwired: 1 in, 1 out]
      }
      n102 = node-c288(w11) -> ()  [unwired: 1 out]
    }
    frame Error {
    }
  }
  "error out" <- w4
